vi "ExposeMapperUpdateValue.vi"(8 "Allow Variant Values (f)":bool, 10 "Namepath Info":T1, 11 "Value In (or type, reference)":refnum<data-value>) -> (1 "Updated controls":refnum<vi>[](array[refnum]), 3 "Value Out Ref":refnum<data-value>)   [LabVIEW 2017]
uses:
  ExposeObjectMapNamepathData.ctl
  ExposeMapperDataTypeEnum.ctl
  ExposeObjectMapContainerTypeEnum.ctl
  ExposeMapperUpdateNamepathPartDescriptorEnum.ctl
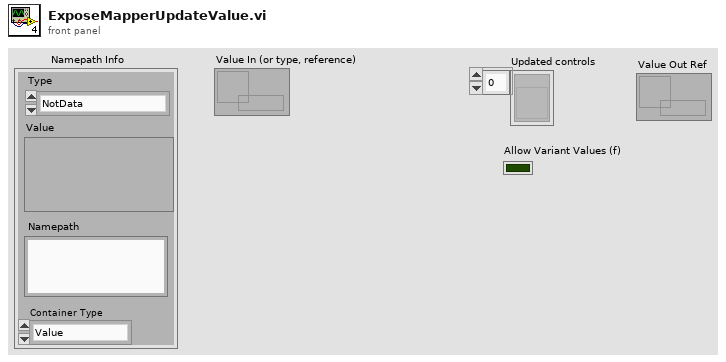
[diagram p1: front panel]
types:
  T1 = typedef "ExposeObjectMapNamepathData.ctl" = cluster{"Type":T2, "Value":variant, "Namepath":string, "Container Type":T3}
  T2 = typedef "ExposeMapperDataTypeEnum.ctl" = enum16{"NotData", "int8", "byte", "int16", "uint16", "int32", "uint32", "int64", "uint64", "Single", "Double", "String", "Boolean", "Container"}
  T3 = typedef "ExposeObjectMapContainerTypeEnum.ctl" = enum16{"Value", "Array", "Waveform", "NetContainer"}
  T4 = typedef "ExposeMapperUpdateNamepathPartDescriptorEnum.ctl" = enum16{"Invalid (Org. Val))", "Default Value", "Value", "Variant", "Cluster", "Array", "Refnum"}
  T5 = typedef "ExposeMapperUpdateNamepathPartDescriptor.ctl" = cluster{"Parent Type":T4, "Property Name":string, "Element Index":i32, "Control":refnum<vi>, "Value Ref":refnum<data-value>, "Has value ref":bool, "Container Type":T3}
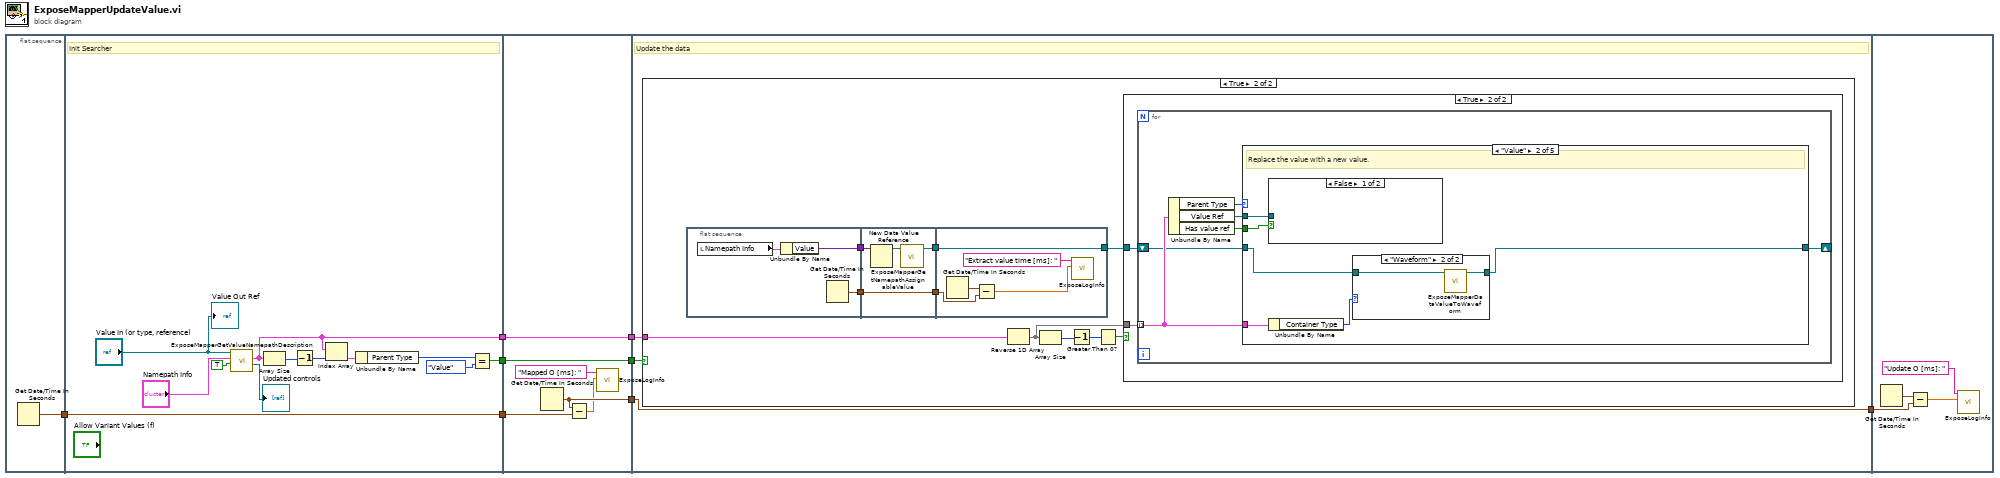
[diagram p0: block diagram]
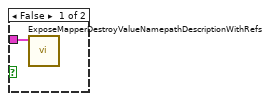
[diagram p2: hidden frame]
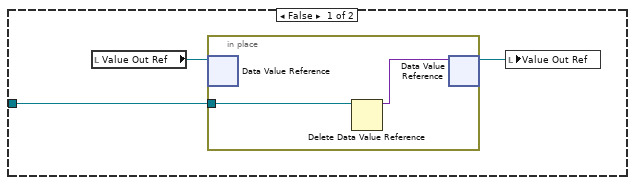
[diagram p3: hidden frame]
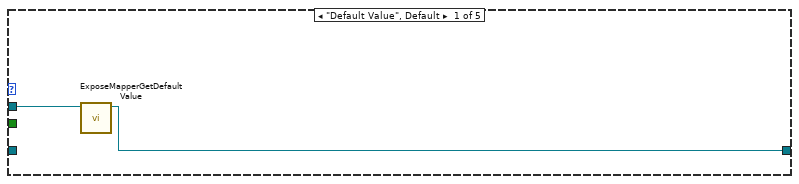
[diagram p4: hidden frame]
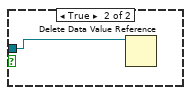
[diagram p6: hidden frame]
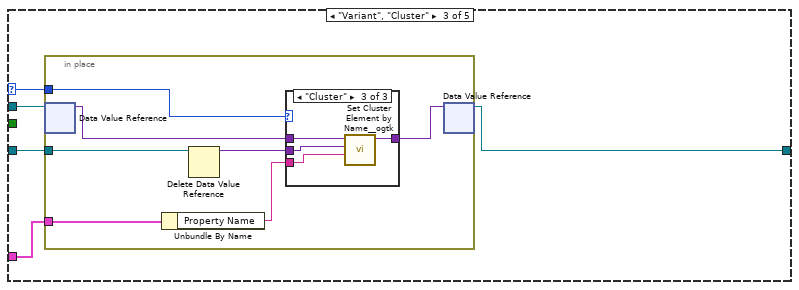
[diagram p7: hidden frame]
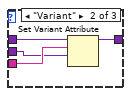
[diagram p9: hidden frame]
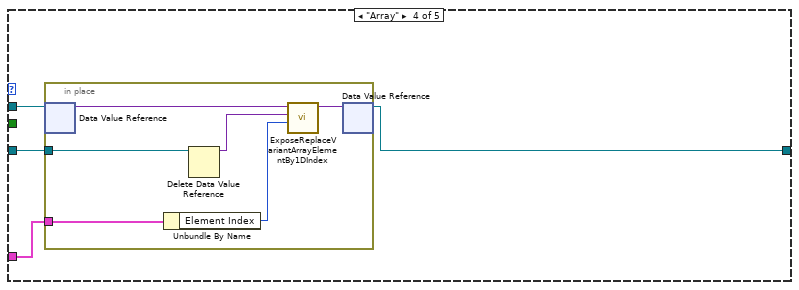
[diagram p10: hidden frame]
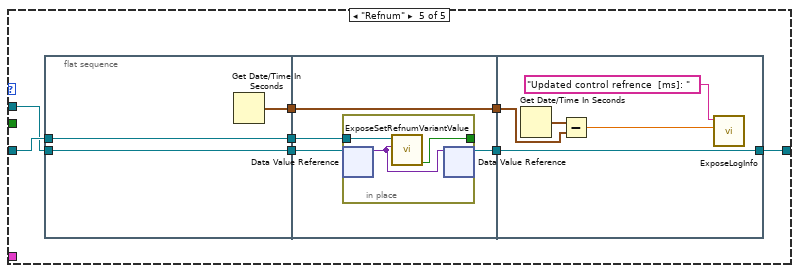
[diagram p11: hidden frame]
diagram:
  n1 = flat-sequence {
    tunnel: [w9] -> w3
    tunnel: [w12] -> w8
    tunnel: [w14] -> w6
    tunnel: [w10] -> w4
    tunnel: w3 -> [w10]
    tunnel: w8 -> [w27]
    tunnel: [w27] -> w7
    tunnel: w6 -> [w26]
    tunnel: [w26] -> w5
    tunnel: w4 -> [w24]
    tunnel: [w25] -> w2
    tunnel: w7 -> [w30]
    tunnel: w5 -> [w29]
    tunnel: w2 -> [w28]
    tunnel: [w28] -> w1
    tunnel: w1 -> [w135]
    frame #0 {
      n2 = Get Date/Time In Seconds() -> (seconds since 1Jan1904=w9:timestamp)
    }
    frame #1 {
      # "Init Searcher"
      n3 = call "ExposeMapperGetValueNamepathDescription.vi"("ColRefVals"=TRUE, "Namepath Info"="Namepath Info", "Data Value Reference in"="Value In (or type, reference)") -> ("Controls Found"=→"Updated controls":refnum<vi>[], "NPDsc"=w12:T5[])  [unwired: 6 in, 1 out]
      n4 = Array Size(array=w12) -> (size(s)=w19:i32)
      n5 = Decrement(x=w19) -> (x-1=w18:i32)
      n6 = Index Array(array=w12, index=w18) -> (element=w17:T5)
      n7 = Unbundle By Name(w17) -> ("Parent Type"=w16:T4)
      n8 = Equal?(x=w16, y=ExposeMapperUpdateNamepathPartDescriptorEnum."Value") -> (x = y?=w14:bool)
      "Value Out Ref" <- "Value In (or type, reference)"
    }
    frame #2 {
      n9 = Get Date/Time In Seconds() -> (seconds since 1Jan1904=w25:timestamp)
      n10 = Subtract(x=w25, y=w24) -> (x-y=w22:dbl)
      n11 = call "ExposeLogInfo.vi"("Action time [ms]"=w22, "message"="Mapped O [ms]: " ("string")) -> ()  [unwired: 10 in]
    }
    frame #3 {
      # "Update the data"
      n12 = case shown="True" w29 {
        tunnel: w30 -> [w31 w34]
        frame False {
          n13 = call "ExposeMapperDestroyValueNamepathDescriptionWithRefs.vi"("NPDsc"=w31) -> ()  [unwired: 10 in, 1 out]
        }
        frame True {
          n14 = flat-sequence {
            tunnel: [w123] -> w41
            tunnel: [w121] -> w37
            tunnel: [w127] -> w40
            tunnel: w41 -> [w127]
            tunnel: [w125] -> w39
            tunnel: w37 -> [w124]
            tunnel: [w128] -> w38
            tunnel: w40 -> [w129]
            tunnel: w39 -> [w128]
            frame #0 {
              n15 = local read "Namepath Info"() -> (w122:T1)
              n16 = Unbundle By Name(w122) -> ("Value"=w121:variant)
              n17 = Get Date/Time In Seconds() -> (seconds since 1Jan1904=w123:timestamp)
            }
            frame #1 {
              n18 = New Data Value Reference(data value=w124) -> (data value reference=w126:refnum<data-value>)  [unwired: 1 in, 1 out]
              n19 = call "ExposeMapperGetNamepathAssignableValue.vi"("Data Val Ref in"=w126) -> ("Data Val Ref Out"=w125:refnum<data-value>)  [unwired: 10 in]
            }
            frame #2 {
              n20 = Get Date/Time In Seconds() -> (seconds since 1Jan1904=w132:timestamp)
              n21 = Subtract(x=w132, y=w129) -> (x-y=w130:dbl)
              n22 = call "ExposeLogInfo.vi"("Action time [ms]"=w130, "message"="Extract value time [ms]: " ("string")) -> ()  [unwired: 10 in]
            }
          }
          n23 = Reverse 1D Array(array=w34) -> (reversed array=w33:T5[])
          n24 = Array Size(array=w33) -> (size(s)=w36:i32)
          n25 = Decrement(x=w36) -> (x-1=w32:i32)
          n26 = Greater Than 0?(x=w32) -> (x > 0?=w35:bool)
          n27 = case shown="True" w35 {
            tunnel: w38 -> [w43 w47]
            tunnel: w33 -> [_ w48]
            frame False {
              n28 = local read "Value Out Ref"() -> (w44:refnum<data-value>)
              n29 = in-place {
                in-place-border: w43 -> [w46]
                n30 = in-place-dvr #1(w44) -> ()  [unwired: 2 out]
                n31 = Delete Data Value Reference(data value reference=w46) -> (data value=w45:variant)  [unwired: 1 in, 1 out]
                n32 = in-place-dvr #1(w45) -> (w42:refnum<data-value>)  [unwired: 1 out]
              }
              n33 = local write "Value Out Ref"(w42) -> ()
            }
            frame True {
              n34 = for {
                tunnel: w48 -> [w53] mode=indexing
                shift-right: [w51] -> _
                shift-left: w47 -> [w49]
                n35 = Unbundle By Name(w53) -> ("Parent Type"=w54:T4, "Value Ref"=w52:refnum<data-value>, "Has value ref"=w50:bool)
                n36 = case shown="\"Value\"" w54 {
                  selector: w54 -> [_ _ w69 _ _]
                  tunnel: w53 -> [_ w60 w70 w89 _]
                  tunnel: w52 -> [w56 w62 w71 w90 w104]
                  tunnel: [w55 w57 w68 w88 w98] -> w51
                  tunnel: w49 -> [_ w58 w67 w91 w105]
                  tunnel: w50 -> [_ w61 _ _ _]
                  frame "Default Value", Default {
                    n37 = call "ExposeMapperGetDefaultValue.vi"("Data Val Ref in"=w56) -> ("Data Val Ref Out"=w55:refnum<data-value>)  [unwired: 10 in]
                  }
                  frame "Value" {
                    # "Replace the value with a new value."
                    n38 = case shown="False" w61 {
                      tunnel: w62 -> [_ w66]
                      frame False {
                      }
                      frame True {
                        n39 = Delete Data Value Reference(data value reference=w66) -> ()  [unwired: 1 in, 2 out]
                      }
                    }
                    n40 = Unbundle By Name(w60) -> ("Container Type"=w59:T3)
                    n41 = case shown="\"Waveform\"" w59 {
                      tunnel: w58 -> [w63 w65]
                      tunnel: [w63 w64] -> w57
                      frame "Value", Default {
                      }
                      frame "Waveform" {
                        n42 = call "ExposeMapperDataValueToWaveform.vi"("Data Value Reference in"=w65) -> ("Data Value Reference out"=w64:refnum<data-value>)  [unwired: 10 in]
                      }
                    }
                  }
                  frame "Variant", "Cluster" {
                    n43 = in-place {
                      in-place-border: w70 -> [w78]
                      in-place-border: w69 -> [w77]
                      in-place-border: w67 -> [w73]
                      n44 = in-place-dvr #2(w71) -> (w76:variant)  [unwired: 1 out]
                      n45 = Unbundle By Name(w78) -> ("Property Name"=w75:string)
                      n46 = Delete Data Value Reference(data value reference=w73) -> (data value=w72:variant)  [unwired: 1 in, 1 out]
                      n47 = case shown="\"Cluster\"" w77 {
                        tunnel: w76 -> [w79 w83 w87]
                        tunnel: [w79 w81 w85] -> w74
                        tunnel: w75 -> [_ w82 w86]
                        tunnel: w72 -> [_ w80 w84]
                        frame Default {
                        }
                        frame "Variant" {
                          n48 = Set Variant Attribute(Variant=w83, name=w82, value=w80) -> (Variant out=w81:variant)  [unwired: 1 in, 2 out]
                        }
                        frame "Cluster" {
                          n49 = call <userlib>:"Set Cluster Element by Name__ogtk.vi"("Element Name (\"\": New Element Data Name)"=w86, "New Element Value"=w84, "Cluster"=w87) -> ("VCluster out"=w85:variant)  [unwired: 6 in, 2 out]
                        }
                      }
                      n50 = in-place-dvr #2(w74) -> (w68:refnum<data-value>)  [unwired: 1 out]
                    }
                  }
                  frame "Array" {
                    n51 = in-place {
                      in-place-border: w91 -> [w95]
                      in-place-border: w89 -> [w93]
                      n52 = in-place-dvr #3(w90) -> (w97:variant)  [unwired: 1 out]
                      n53 = Unbundle By Name(w93) -> ("Element Index"=w92:i32)
                      n54 = Delete Data Value Reference(data value reference=w95) -> (data value=w94:variant)  [unwired: 1 in, 1 out]
                      n55 = call "ExposeReplaceVariantArrayElementBy1DIndex.vi"("Index (1D)"=w92, "Value"=w94, "Array in"=w97) -> ("Array out"=w96:variant)  [unwired: 8 in]
                      n56 = in-place-dvr #3(w96) -> (w88:refnum<data-value>)  [unwired: 1 out]
                    }
                  }
                  frame "Refnum" {
                    n57 = flat-sequence {
                      tunnel: w104 -> [w107]
                      tunnel: w105 -> [w108]
                      tunnel: [w108] -> w103
                      tunnel: [w107] -> w102
                      tunnel: [w106] -> w100
                      tunnel: w103 -> [w109]
                      tunnel: w102 -> [w111]
                      tunnel: [w112] -> w101
                      tunnel: w100 -> [w112]
                      tunnel: [w110] -> w99
                      tunnel: w101 -> [w117]
                      tunnel: w99 -> [w116]
                      tunnel: [w116] -> w98
                      frame #0 {
                        n58 = Get Date/Time In Seconds() -> (seconds since 1Jan1904=w106:timestamp)
                      }
                      frame #1 {
                        n59 = in-place {
                          in-place-border: w109 -> [w114]
                          in-place-border: [w113] -> _
                          n60 = in-place-dvr #4(w111) -> (w115:variant)  [unwired: 1 out]
                          n61 = call "ExposeSetRefnumVariantValue.vi"("Control"=w115, "Value In (reference)"=w114) -> ("IsControl"=w113:bool)  [unwired: 9 in]
                          n62 = in-place-dvr #4(w115) -> (w110:refnum<data-value>)  [unwired: 1 out]
                        }
                      }
                      frame #2 {
                        n63 = Get Date/Time In Seconds() -> (seconds since 1Jan1904=w120:timestamp)
                        n64 = Subtract(x=w120, y=w117) -> (x-y=w118:dbl)
                        n65 = call "ExposeLogInfo.vi"("Action time [ms]"=w118, "message"="Updated control refrence  [ms]: " ("string")) -> ()  [unwired: 10 in]
                      }
                    }
                  }
                }
              }
            }
          }
        }
      }
    }
    frame #4 {
      n66 = Get Date/Time In Seconds() -> (seconds since 1Jan1904=w136:timestamp)
      n67 = Subtract(x=w136, y=w135) -> (x-y=w133:dbl)
      n68 = call "ExposeLogInfo.vi"("Action time [ms]"=w133, "message"="Update O [ms]: " ("string")) -> ()  [unwired: 10 in]
    }
  }
